vi "MHTML Image Section.vi"(4 "Boundary (\"\")":string, 5 "error in (no error)":errorcluster, 8 "image data":T1) -> (0 "error out":errorcluster, 2 "Image Tag":string, 3 "MIME Image":string)   [LabVIEW 2011]
uses:
  <vilib>/picture/picture.llb/imagedata.ctl
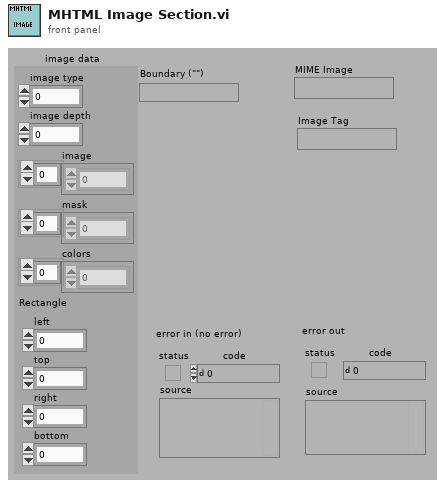
[diagram p1: front panel]
types:
  T1 = typedef "imagedata.ctl" = cluster{"image type":i32, "image depth":i32, "image":u8[], "mask":u8[], "colors":u32[], "Rectangle":cluster{"left":i16, "top":i16, "right":i16, "bottom":i16}}
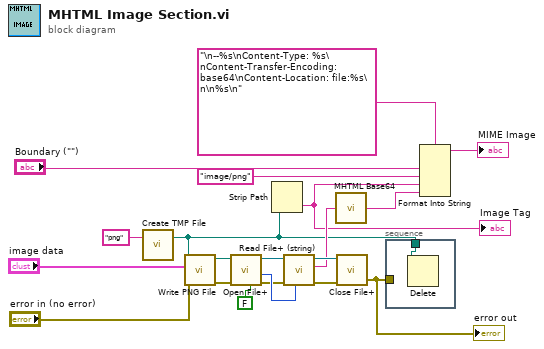
[diagram p0: block diagram]
diagram:
  n1 = call "Create TMP File.vi"("PrefixString(\"xxx\")"="png" ("PrefixString(\"xxx\")")) -> ("Path"=w7:path)  [unwired: 2 out]
  n2 = call <vilib>:"Write PNG File.vi"("error in (no error)"="error in (no error)", "image data"="image data", "path to PNG file"=w7) -> ("error out"=w12:errorcluster, "path"=w11:path)  [unwired: 7 out]
  n3 = call <vilib>:"Open File+.vi"("advisory dialog? (display:T)"=FALSE, "error in (not an error)"=w12, "file path (\" \")"=w11) -> ("error out"=w15:errorcluster, "file size (bytes)"=w16:i32, "refnum"=w17:refnum<file>)  [unwired: 4 in, 2 out]
  n4 = Strip Path(path=w7) -> (name=w2:string)  [unwired: 1 out]
  "Image Tag" <- w2
  n5 = call <vilib>:"Read File+ (string).vi"("count"=w16, "error in (no error)"=w15, "refnum"=w17) -> ("error out"=w13:errorcluster, "string"=w10:string, "dup refnum"=w14:refnum<file>)  [unwired: 2 in, 4 out]
  n6 = call "MHTML Base64.vi"("Binary String"=w10) -> ("String (Base64)"=w6:string)  [unwired: 14 out]
  n7 = call <vilib>:"Close File+.vi"("error in (no error)"=w13, "refnum"=w14) -> ("error out"=w1:errorcluster)  [unwired: 5 out]
  "error out" <- w1
  n8 = stacked-sequence {
    tunnel: w7 -> [w21]
    tunnel: w1 -> [_]
    frame #0 {
      n9 = Delete(path (use dialog)=w21) -> ()  [unwired: 1 in, 6 out]
    }
  }
  n10 = Format Into String(format string="\n--%s\nContent-Type: %s\nContent-Transfer-Encoding: base64\nContent-Location: file:%s\n\n%s\n", "Boundary (\"\")", "image/png", w2, w6) -> (resulting string=→"MIME Image":string)  [unwired: 2 in, 1 out]
